vi "FlatToRichnidaqmx_grpc_CfgImplicitTimingRequest.vi"(5 "OutputClusterType":T1, 11 "InputCluster":T3) -> (3 "OutputCluster":T1)   [LabVIEW 2021, in "NI_DAQmx_client.lvlib"]
uses:
  NI_DAQmx_client.lvlib
  nidaqmx_grpc_CfgImplicitTimingRequest_sample_mode_enum/nidaqmx_grpc_CfgImplicitTimingRequest_sample_mode_enum.lvclass
  nidevice_grpc_Session_session/nidevice_grpc_Session_session.lvclass
  nidevice_grpc_Session.ctl
  nidaqmx_grpc_CfgImplicitTimingRequest.ctl
  nidaqmx_grpc_AcquisitionType.ctl
  nidevice_grpc_Session_Flat.ctl
  nidaqmx_grpc_CfgImplicitTimingRequest_Flat.ctl
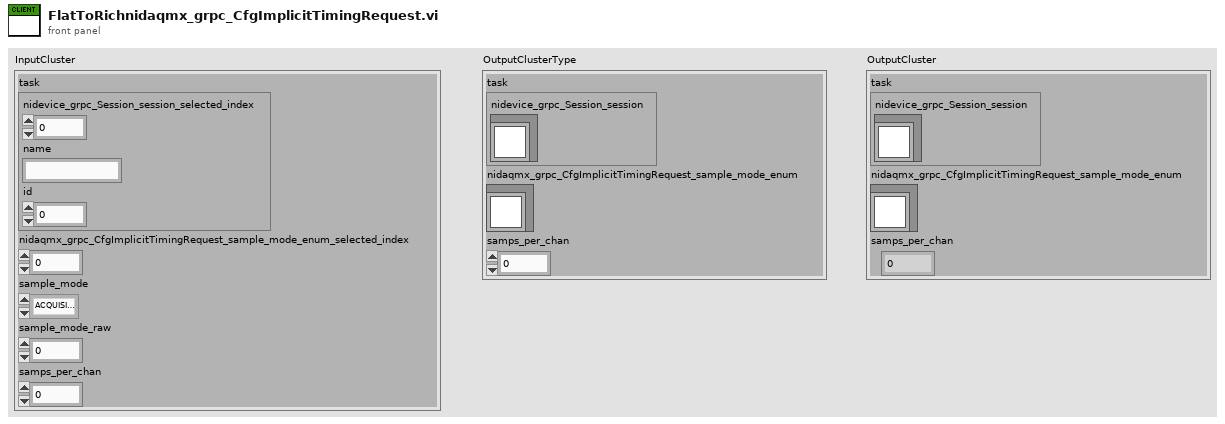
[diagram p1: front panel]
types:
  T1 = typedef "NI_DAQmx_client.lvlib/nidaqmx_grpc_CfgImplicitTimingRequest.ctl" = cluster{"task":T2, "nidaqmx_grpc_CfgImplicitTimingRequest_sample_mode_enum":refnum<class "nidaqmx_grpc_CfgImplicitTimingRequest_sample_mode_enum.lvclass">, "samps_per_chan":u64}
  T2 = typedef "NI_DAQmx_client.lvlib/nidevice_grpc_Session.ctl" = cluster{"nidevice_grpc_Session_session":refnum<class "nidevice_grpc_Session_session.lvclass">}
  T3 = typedef "NI_DAQmx_client.lvlib/nidaqmx_grpc_CfgImplicitTimingRequest_Flat.ctl" = cluster{"task":T4, "nidaqmx_grpc_CfgImplicitTimingRequest_sample_mode_enum_selected_index":i32, "sample_mode":T5, "sample_mode_raw":i32, "samps_per_chan":u64}
  T4 = typedef "NI_DAQmx_client.lvlib/nidevice_grpc_Session_Flat.ctl" = cluster{"nidevice_grpc_Session_session_selected_index":i32, "name":string, "id":u32}
  T5 = typedef "NI_DAQmx_client.lvlib/nidaqmx_grpc_AcquisitionType.ctl" = enum32{"ACQUISITION_TYPE_UNSPECIFIED", "ACQUISITION_TYPE_FINITE_SAMPS", "ACQUISITION_TYPE_CONT_SAMPS", "ACQUISITION_TYPE_HW_TIMED_SINGLE_POINT"}
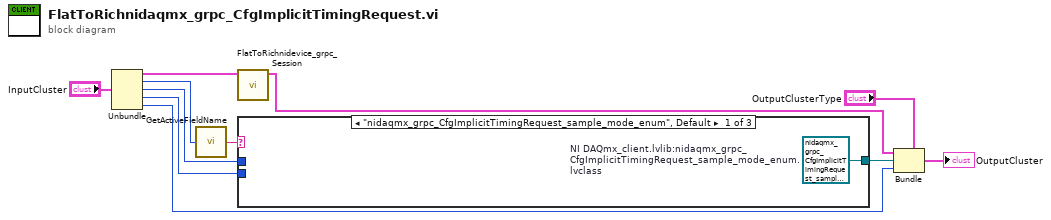
[diagram p0: block diagram]
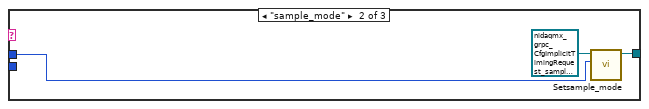
[diagram p2: hidden frame]
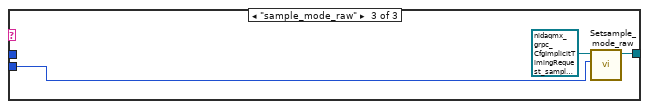
[diagram p3: hidden frame]
diagram:
  n1 = Unbundle "Unbundle"("InputCluster") -> ("task"=w8:T4, "nidaqmx_grpc_CfgImplicitTimingRequest_sample_mode_enum_selected_index"=w6:i32, "sample_mode"=w3:T5, "sample_mode_raw"=w2:i32, "samps_per_chan"=w1:u64)
  n2 = call "GetActiveFieldName.vi"("protobuf index"=w6) -> ("oneof field name"=w5:string)
  n3 = call "FlatToRichnidevice_grpc_Session.vi"("InputCluster"=w8) -> ("OutputCluster"=w7:T2)  [unwired: 10 in]
  n4 = case "nidaqmx_grpc_CfgImplicitTimingRequest_sample_mode_enum" shown="\"nidaqmx_grpc_CfgImplicitTimingRequest_sample_mode_enum\", Default" w5 {
    tunnel: [w12 w14 w17] -> w4
    tunnel: w3 -> [_ w15 _]
    tunnel: w2 -> [_ _ w18]
    frame "nidaqmx_grpc_CfgImplicitTimingRequest_sample_mode_enum", Default {
      w12 = refnum<class "nidaqmx_grpc_CfgImplicitTimingRequest_sample_mode_enum.lvclass"> refnum  # NI DAQmx_client.lvlib:nidaqmx_grpc_CfgImplicitTimingRequest_sample_mode_enum.lvclass
    }
    frame "sample_mode" {
      n5 = call "Setsample_mode.vi"("Set_Val"=w15, "OneOfTemplate in"=refnum<class "nidaqmx_grpc_CfgImplicitTimingRequest_sample_mode_enum.lvclass"> refnum) -> ("OneOfTemplate out"=w14:refnum<class "nidaqmx_grpc_CfgImplicitTimingRequest_sample_mode_enum.lvclass">)  [unwired: 8 in, 1 out]
    }
    frame "sample_mode_raw" {
      n6 = call "Setsample_mode_raw.vi"("Set_Val"=w18, "OneOfTemplate in"=refnum<class "nidaqmx_grpc_CfgImplicitTimingRequest_sample_mode_enum.lvclass"> refnum) -> ("OneOfTemplate out"=w17:refnum<class "nidaqmx_grpc_CfgImplicitTimingRequest_sample_mode_enum.lvclass">)  [unwired: 8 in, 1 out]
    }
  }
  n7 = Bundle "Bundle"(cluster="OutputClusterType", "task"=w7, "nidaqmx_grpc_CfgImplicitTimingRequest_sample_mode_enum"=w4, "samps_per_chan"=w1) -> (→"OutputCluster":T1)
